vi "NavX Tester.vi"() -> ()   [LabVIEW 2018]
doc: "This VI implements the framework and scheduler for your robotics program. It should not be necessary to modify the framework. You are expected to add your code to the VIs called from Robot Main - the ones located in the Team Code folder within the project."
uses:
  <vilib>/Rock Robotics/WPI/ThirdParty/Sensors/navX/_TypeDefs/Z900_navX_SerialStreamTypeDef.ctl
  <vilib>/Rock Robotics/WPI/ThirdParty/Sensors/navX/_TypeDefs/Flags/Z900_navX_Flags_OpStatusTypeDef.ctl
  <vilib>/Rock Robotics/WPI/ThirdParty/Sensors/navX/_TypeDefs/Flags/Z900_navX_Flags_CalibrationStatusTypeDef.ctl
  <vilib>/Rock Robotics/WPI/ThirdParty/Sensors/navX/_TypeDefs/Flags/Z900_navX_Flags_HardwareRevTypeDef.ctl
  <vilib>/Rock Robotics/WPI/ThirdParty/Sensors/navX/_TypeDefs/Flags/Z900_navX_Flags_OmnimountConfigTypeDef.ctl
  <vilib>/Rock Robotics/WPI/ThirdParty/Sensors/navX/_TypeDefs/FRIC_navX_TestStatesTypeDef_I2C.ctl
  <vilib>/Rock Robotics/WPI/ThirdParty/Sensors/navX/_TypeDefs/FRIC_navX_DeviceNumbersTypeDef.ctl
  <vilib>/Rock Robotics/WPI/ThirdParty/Sensors/navX/_Processing Loop/FRIC_navX_Internal_SPI_ProcessingLoop.vi
  <vilib>/Rock Robotics/WPI/ThirdParty/Sensors/navX/_Processing Loop/FRIC_navX_Internal_I2C_ProcessingLoop.vi
  <vilib>/Rock Robotics/WPI/ThirdParty/Sensors/navX/_Processing Loop/FRIC_navX_Internal_Serial_ProcessingLoop.vi
  <vilib>/Rock Robotics/WPI/ThirdParty/Sensors/navX/_Processing Loop/FRIC_navX_Internal_USB_ProcessingLoop.vi
panel:
  in  "Tab Control":enum32{"Device 0", "Device 1"}(tab)
  out "String":string
  in  "Next":bool
  in  "Exit":bool
  out "Warning":bool
  in  "Change Serial Stream":bool
  out "Connected":bool
  out "Displacement":T1 {"Velocity X" format="%.8f"; "Velocity Y" format="%.8f"; "Velocity Z" format="%.8f"; "Displace X" format="%.8f"; "Displace Y" format="%.8f"; "Displace Z" format="%.8f"}
  out "MPUTemp":dbl format="%.2f"
  out "Board Information":T4 {"Board"."Hardware Revision" items=["navX-MXP"=33, "navX-Micro"=40]; "Omnimount Config" items=["DEFAULT", "X_UP", "X_DOWN", "Y_UP", "Y_DOWN", "Z_UP", "Z_DOWN"]}
  out "Linear Acceleration":cluster{"X":dbl, "Y":dbl, "Z":dbl} {"X" format="%.6f"; "Y" format="%.6f"; "Z" format="%.6f"}
  out "Quaternion":T5 {"Quat W" format="%.8f"; "Quat X" format="%.8f"; "Quat Y" format="%.8f"; "Quat Z" format="%.8f"}
  out "Status":T8 {"OP Status" items=["INITIALIZING", "SELFTEST_IN_PROGRESS", "ERROR", "IMU_AUTOCAL_IN_PROGRESS", "NORMAL"]; "Calibration Status" items=["IMU_CAL_STATE_MASK"=3, "IMU_CAL_STATE_INPROGRESS"=0, "IMU_CAL_STATE_ACCUMULATE"=1, "IMU_CAL_STATE_COMPLETE"=2]}
  out "YRPHfH":T9 {"Yaw" format="%.2f"; "Roll" format="%.2f"; "Pitch" format="%.2f"; "Heading" format="%.2f"; "Fused Heading" format="%.2f"}
  out "Timestamp":u32
  out "Error":bool
  out "error":errorcluster
  in  "Zero Yaw":bool
  in  "Zero Displacement":bool
  in  "Zero Velocity":bool
  out "Raw Values":T10 {"Accel X" format="%.8f"; "Accel Y" format="%.8f"; "Accel Z" format="%.8f"; "Gyro X" format="%.8f"; "Gyro Y" format="%.8f"; "Gyro Z" format="%.8f"; "Mag X" format="%.8f"; "Mag Y" format="%.8f"; "Mag Z" format="%.8f"}
  in  "Stream Type":T11=enum."AHRSAndPositioning"
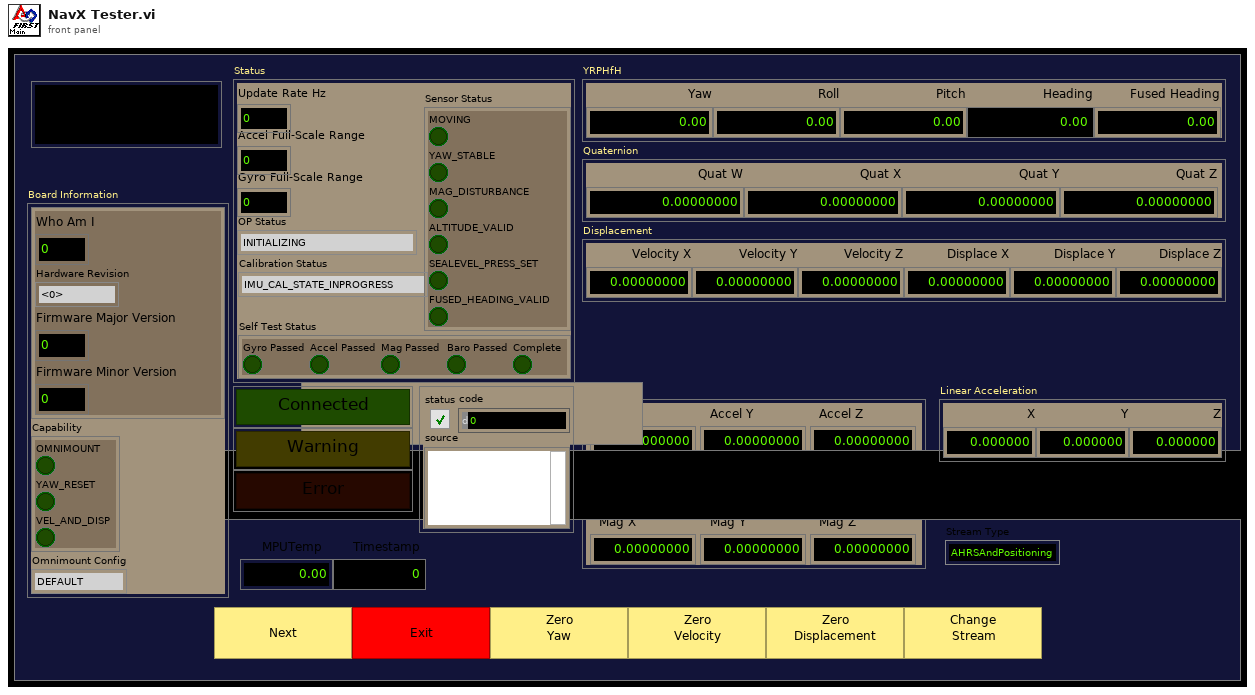
[diagram p1: front panel]
types:
  T1 = cluster{"Velocity X":dbl, "Velocity Y":dbl, "Velocity Z":dbl, "Displace X":dbl, "Displace Y":dbl, "Displace Z":dbl}
  T2 = typedef "Z900_navX_Flags_HardwareRevTypeDef.ctl" = u8
  T3 = typedef "Z900_navX_Flags_OmnimountConfigTypeDef.ctl" = u8
  T4 = cluster{"Board":cluster{"Who Am I":u8, "Hardware Revision":T2, "Firmware Major Version":u8, "Firmware Minor Version":u8}, "Capability":cluster{"OMNIMOUNT":bool, "YAW_RESET":bool, "VEL_AND_DISP":bool}, "Omnimount Config":T3}
  T5 = cluster{"Quat W":dbl, "Quat X":dbl, "Quat Y":dbl, "Quat Z":dbl}
  T6 = typedef "Z900_navX_Flags_OpStatusTypeDef.ctl" = u8
  T7 = typedef "Z900_navX_Flags_CalibrationStatusTypeDef.ctl" = u8
  T8 = cluster{"Update Rate Hz":u8, "Accel Full-Scale Range":u8, "Gyro Full-Scale Range":u16, "OP Status":T6, "Calibration Status":T7, "Sensor Status":cluster{"MOVING":bool, "YAW_STABLE":bool, "MAG_DISTURBANCE":bool, "ALTITUDE_VALID":bool, "SEALEVEL_PRESS_SET":bool, "FUSED_HEADING_VALID":bool}, "Self Test Status":cluster{"Gyro Passed":bool, "Accel Passed":bool, "Mag Passed":bool, "Baro Passed":bool, "Complete":bool}}
  T9 = cluster{"Yaw":dbl, "Roll":dbl, "Pitch":dbl, "Heading":dbl, "Fused Heading":dbl}
  T10 = cluster{"Accel X":dbl, "Accel Y":dbl, "Accel Z":dbl, "Gyro X":dbl, "Gyro Y":dbl, "Gyro Z":dbl, "Mag X":dbl, "Mag Y":dbl, "Mag Z":dbl}
  T11 = typedef "Z900_navX_SerialStreamTypeDef.ctl" = enum16{"YRPH", "Quaterinons", "Gyro/Raw", "AHRS", "AHRSAndPositioning", "AHRSAndPOSTime"}
  T12 = typedef "FRIC_navX_TestStatesTypeDef_I2C.ctl" = enum16{"Unknown", "Start SPI", "Start I2C", "Start Serial", "Start USB", "Hault", "Exit"}
  T13 = typedef "FRIC_navX_DeviceNumbersTypeDef.ctl" = enum16{"Dev0", "Dev1", "Dev2", "Dev3"}
  T14 = cluster{"Velocity X":dbl, "Velocity Y":dbl, "Velocity Z":dbl, "Displacement X":dbl, "Displacement Y":dbl, "Displacement Z":dbl}
  T15 = cluster{"LinearAcceleration X":dbl, "LinearAcceleration Y":dbl, "LinearAcceleration Z":dbl}
  T16 = cluster{"Update Rate Hz":u8, "Accelerometer Full-Scale Range":u8, "Gyro Full-Scale Range":u16, "OP Status":T6, "Calibration Status":T7, "Sensor Status":cluster{"MOVING":bool, "YAW_STABLE":bool, "MAG_DISTURBANCE":bool, "ALTITUDE_VALID":bool, "SEALEVEL_PRESS_SET":bool, "FUSED_HEADING_VALID":bool}, "Self Test Status":cluster{"Gyro Passed":bool, "Accel Passed":bool, "Mag Passed":bool, "Baro Passed":bool, "Complete":bool}}
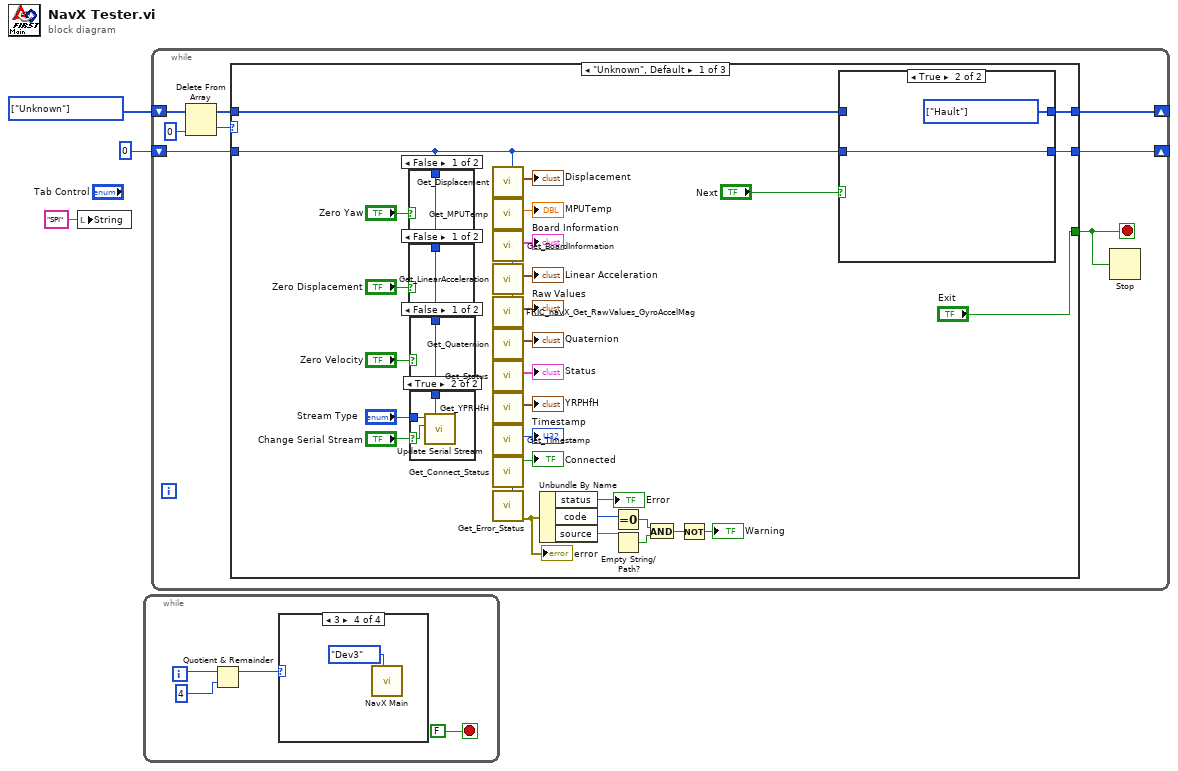
[diagram p0: block diagram]
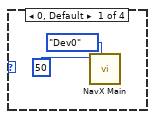
[diagram p2: hidden frame]
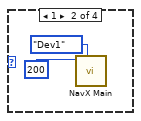
[diagram p3: hidden frame]
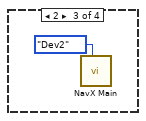
[diagram p4: hidden frame]
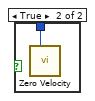
[diagram p7: hidden frame]
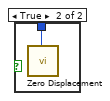
[diagram p8: hidden frame]
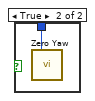
[diagram p9: hidden frame]
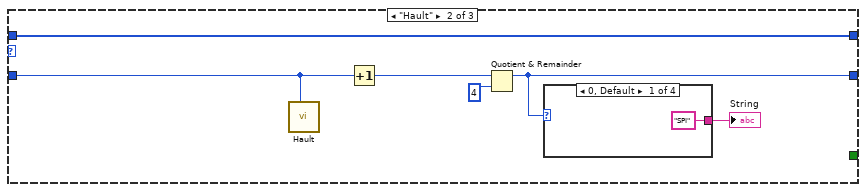
[diagram p10: hidden frame]
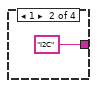
[diagram p11: hidden frame]
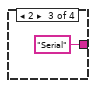
[diagram p12: hidden frame]
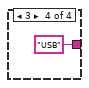
[diagram p13: hidden frame]
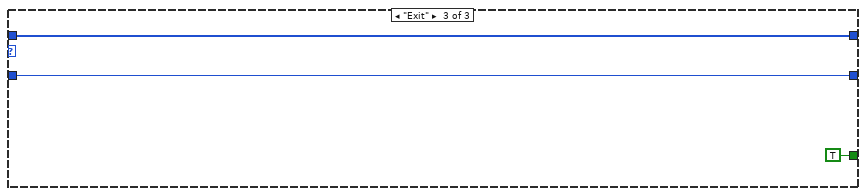
[diagram p14: hidden frame]
diagram:
  w3 = T12[] [enum."Unknown"] items=["Unknown", "Start SPI", "Start I2C", "Start Serial", "Start USB", "Hault", "Exit"]
  n1 = local write "String"("SPI" ("String")) -> ()
  n2 = while {
    i -> [w4]
    stop <- FALSE stop-if-true
    n3 = Quotient & Remainder(x=w4, y=4 ("x")) -> (x-y*floor(x/y)=w7:i32)  [unwired: 1 out]
    n4 = case shown="3" w7 {
      frame 0, Default {
        n5 = call-poly <vilib>:"NavX Main.vi"("Device Number"=FRIC_navX_DeviceNumbersTypeDef."Dev0", "Rate (4Hz-200Hz)"=50) -> ()  [unwired: 10 in]
      }
      frame 1 {
        n6 = call-poly <vilib>:"NavX Main.vi"("Device Number"=FRIC_navX_DeviceNumbersTypeDef."Dev1", "Rate (4Hz-200Hz)"=200) -> ()  [unwired: 10 in]
      }
      frame 2 {
        n7 = call-poly <vilib>:"NavX Main.vi"("Device Number"=FRIC_navX_DeviceNumbersTypeDef."Dev2") -> ()  [unwired: 11 in]
      }
      frame 3 {
        n8 = call-poly <vilib>:"NavX Main.vi"("Device Number"=FRIC_navX_DeviceNumbersTypeDef."Dev3") -> ()  [unwired: 11 in]
      }
    }
  }
  n9 = while "Scheduling loop" {
    shift-right: [w17] -> _
    shift-left: w3 -> [w21]
    shift-right: [w16] -> _
    shift-left: 0 -> [w15]
    stop <- w14 stop-if-true
    n10 = Delete From Array(array=w21, index=0) -> (deleted portion=w19:T12, array with subset deleted=w18:T12[])  [unwired: 1 in]
    n11 = case shown="\"Unknown\", Default" w19 {
      tunnel: ["Exit" _ TRUE] -> w14
      tunnel: w18 -> [w27 w66 w72]
      tunnel: [w26 w66 w72] -> w17
      tunnel: [w24 w61 w71] -> w16
      tunnel: w15 -> [w23 w63 w71]
      frame "Unknown", Default {
        n12 = case shown="False" "Zero Yaw" {
          tunnel: w23 -> [_ w60]
          frame False {
          }
          frame True {
            n13 = call <vilib>:"Zero Yaw.vi"("Device Number"=w60) -> ()  [unwired: 11 in]
          }
        }
        n14 = case shown="False" "Zero Displacement" {
          tunnel: w23 -> [_ w59]
          frame False {
          }
          frame True {
            n15 = call <vilib>:"Zero Displacement.vi"("Device Number"=w59) -> ()  [unwired: 11 in]
          }
        }
        n16 = case shown="False" "Zero Velocity" {
          tunnel: w23 -> [_ w58]
          frame False {
          }
          frame True {
            n17 = call <vilib>:"Zero Velocity.vi"("Device Number"=w58) -> ()  [unwired: 11 in]
          }
        }
        n18 = case shown="True" "Change Serial Stream" {
          selector: "Change Serial Stream" -> [_ w55]
          tunnel: w23 -> [_ w57]
          tunnel: "Stream Type" -> [_ w56]
          frame False {
          }
          frame True {
            n19 = call <vilib>:"Update Serial Stream.vi"("Device Number"=w57, "Update"=w55, "Stream Type"=w56) -> ()  [unwired: 9 in]
          }
        }
        n20 = call <vilib>:"Get_Displacement.vi"("Device Number"=w23) -> ("Displacement"=→"Displacement":T14)  [unwired: 10 in]
        n21 = call <vilib>:"Get_MPUTemp.vi"("Device Number"=w23) -> ("MPUTemp"=→"MPUTemp":dbl)  [unwired: 10 in]
        n22 = call <vilib>:"Get_BoardInformation.vi"("Device Number"=w23) -> ("Board Information"=→"Board Information":T4)  [unwired: 10 in]
        n23 = call <vilib>:"Get_LinearAcceleration.vi"("Device Number"=w23) -> ("Linear Acceleration"=→"Linear Acceleration":T15)  [unwired: 10 in]
        n24 = call <vilib>:"FRIC_navX_Get_RawValues_GyroAccelMag.vi"("Device Number"=w23) -> ("Raw Values (out)"=→"Raw Values":T10)  [unwired: 10 in]
        n25 = call <vilib>:"Get_Quaternion.vi"("Device Number"=w23) -> ("Quaternion"=→"Quaternion":T5)  [unwired: 10 in]
        n26 = call <vilib>:"Get_Status.vi"("Device Number"=w23) -> ("Status"=→"Status":T16)  [unwired: 10 in]
        n27 = call <vilib>:"Get_YPRHfH.vi"("Device Number"=w23) -> ("YRPHfH"=→"YRPHfH":T9)  [unwired: 10 in]
        n28 = call <vilib>:"Get_Timestamp.vi"("Device Number"=w23) -> ("Timestamp"=→"Timestamp":u32)  [unwired: 10 in]
        n29 = call <vilib>:"Get_Connect_Status.vi"("Device Number"=w23) -> ("Connected"=→"Connected":bool)  [unwired: 10 in]
        n30 = call <vilib>:"Get_Error_Status.vi"("Device Number"=w23) -> ("error out"=w43:errorcluster)  [unwired: 10 in]
        "error" <- w43
        n31 = Unbundle By Name(w43) -> ("status"=→"Error":bool, "code"=w45:i32, "source"=w46:string)
        n32 = Equal To 0?(x=w45) -> (x = 0?=w47:bool)
        n33 = Empty String/Path?(string/path=w46) -> (empty?=w48:bool)
        n34 = And(x=w47, y=w48) -> (x .and. y?=w49:bool)
        n35 = Not(x=w49) -> (.not. x?=→"Warning":bool)
        n36 = case shown="True" "Next" {
          tunnel: w27 -> [w52 _]
          tunnel: [w52 w53] -> w26
          tunnel: [w51 w54] -> w24
          tunnel: w23 -> [w51 w54]
          frame False {
          }
          frame True {
            w53 = T12[] [enum."Hault"] items=["Unknown", "Start SPI", "Start I2C", "Start Serial", "Start USB", "Hault", "Exit"]
          }
        }
      }
      frame "Hault" {
        n37 = call <vilib>:"Hault.vi"("Device Number"=w63) -> ()  [unwired: 11 in]
        n38 = Increment(x=w63) -> (x+1=w65:i32)
        n39 = Quotient & Remainder(x=w65, y=4) -> (x-y*floor(x/y)=w61:i32)  [unwired: 1 out]
        n40 = case shown="0, Default" w61 {
          tunnel: ["SPI" ("String") "I2C" ("String") "Serial" ("String") "USB" ("String")] -> w62
          frame 0, Default {
          }
          frame 1 {
          }
          frame 2 {
          }
          frame 3 {
          }
        }
        "String" <- w62
      }
      frame "Exit" {
      }
    }
    n41 = Stop(stop? (T)=w14) -> ()
  }
